vi "Calculate_Desired_Flowrates.vi"(4 "Atmos Pres (mbars)":dbl=1000.0 format="%.2f", 5 "Release temp (deg C)":dbl=20.0 format="%.2f", 6 "Density Ratio":string, 8 "Strength (% by volume)":dbl=3.0 format="%.2f", 9 "Stack Flowrate (l/min)":dbl=20.0 format="%.2f") -> (0 "Error Message":string, 1 "Trace Q l/min":dbl format="%.2f", 2 "Carrier 2 l/min":dbl format="%.2f", 3 "Carrier 1 l/min":dbl format="%.2f")   [LabVIEW 2010]
uses:
  Anemometry/Anemometry Sub Vis/Globals/Gas_management_global.vi
panel:
  # "-Carrier 1 only\n-Carrier 2 only\n-Enter Ratio"
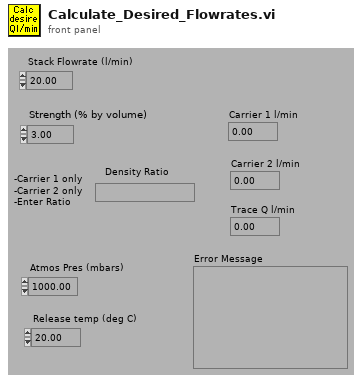
[diagram p1: front panel]
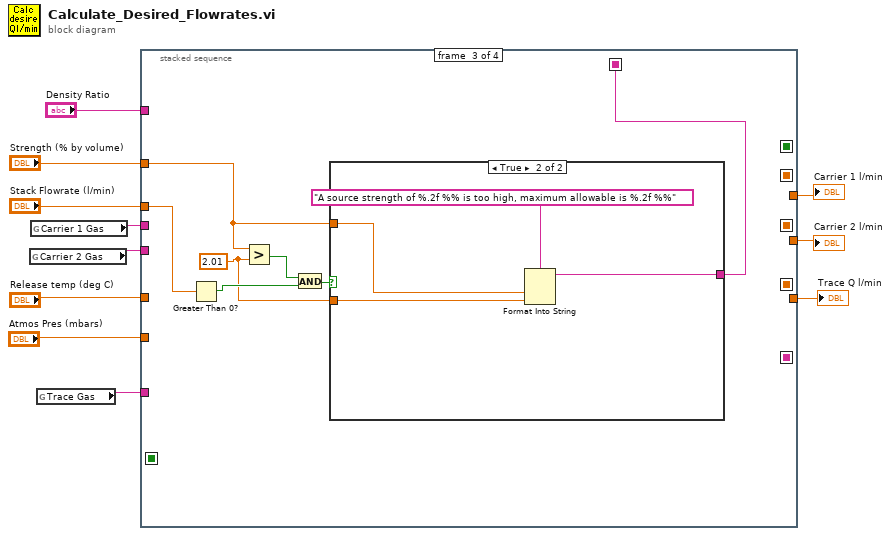
[diagram p0: block diagram]
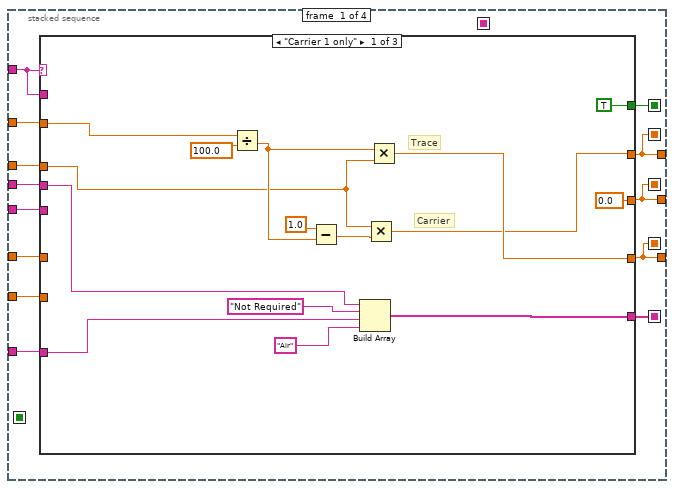
[diagram p2: hidden frame]
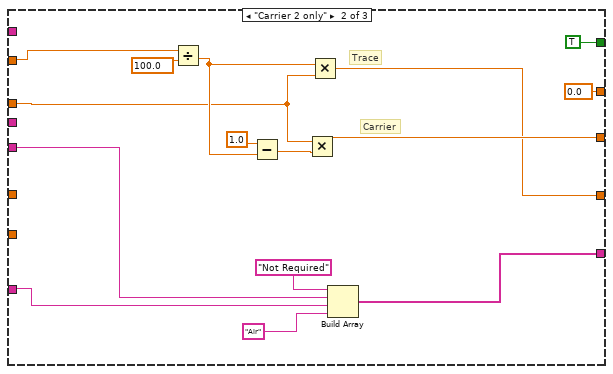
[diagram p3: hidden frame]
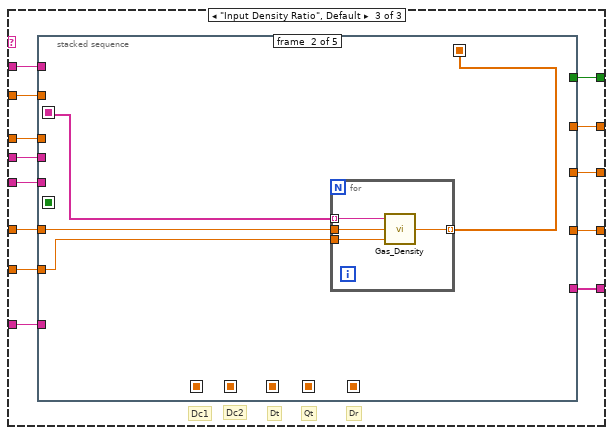
[diagram p4: hidden frame]
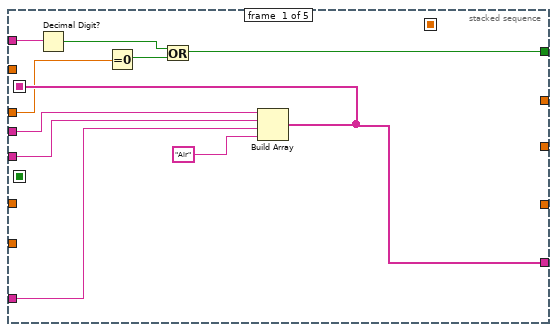
[diagram p5: hidden frame]
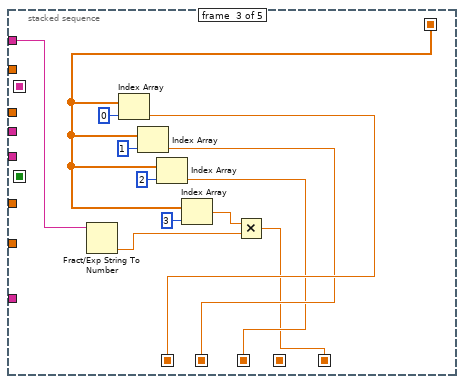
[diagram p6: hidden frame]
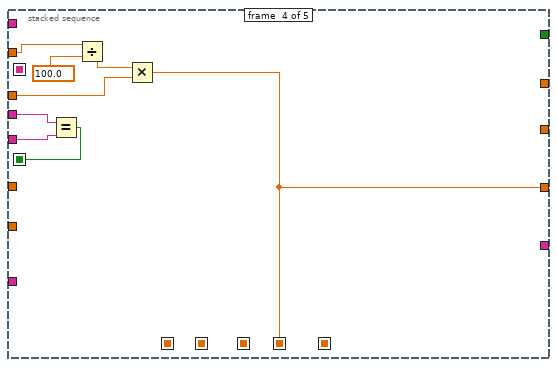
[diagram p7: hidden frame]
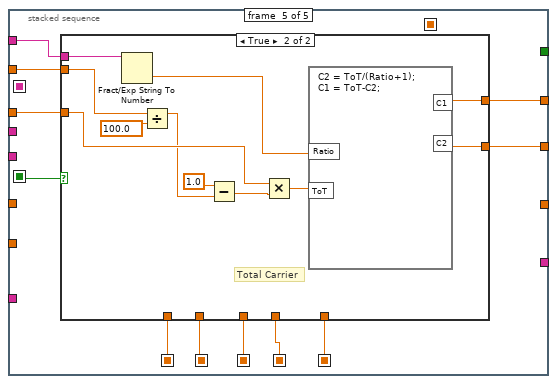
[diagram p8: hidden frame]
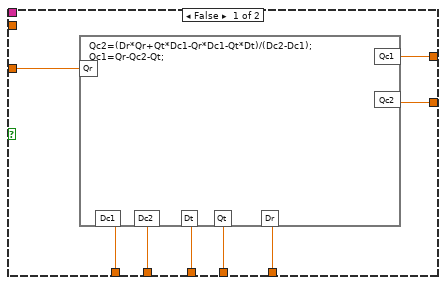
[diagram p9: hidden frame]
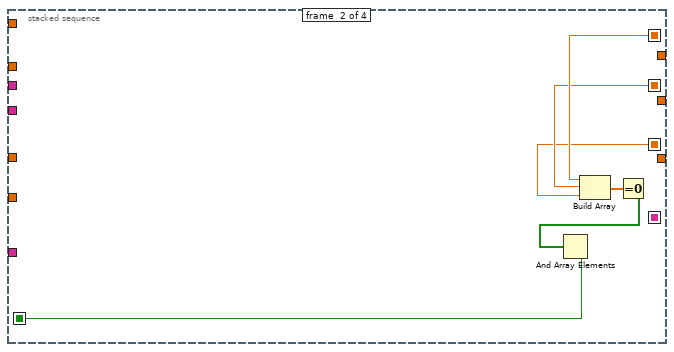
[diagram p10: hidden frame]
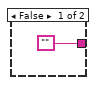
[diagram p11: hidden frame]
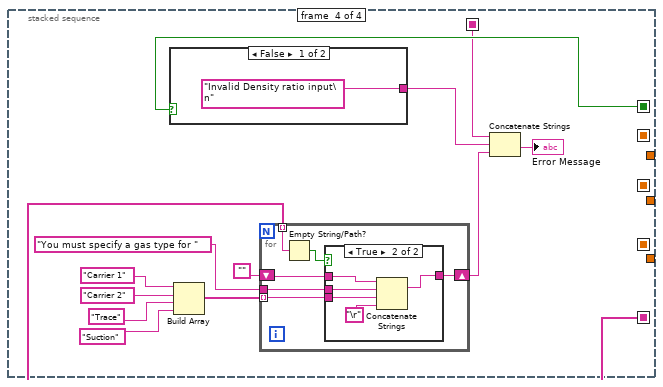
[diagram p12: hidden frame]
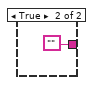
[diagram p13: hidden frame]
diagram:
  n1 = global read "Gas_management_global.vi" "Carrier 2 Gas"() -> (w2:string)
  n2 = global read "Gas_management_global.vi" "Carrier 1 Gas"() -> (w3:string)
  n3 = global read "Gas_management_global.vi" "Trace Gas"() -> (w1:string)
  n4 = stacked-sequence {
    seq-local: [w16 _ _ _] -> [_ _ _ w159]
    seq-local: [w15 _ _ _] -> [_ _ _ w158]
    seq-local: [w12 _ _ _] -> [_ w141 _ _]
    seq-local: [w13 _ _ _] -> [_ w140 _ _]
    seq-local: [w14 _ _ _] -> [_ w139 _ _]
    seq-local: [_ w136 _ _] -> [_ _ _ _]
    seq-local: [_ _ w142 _] -> [_ _ _ w154]
    tunnel: "Release temp (deg C)" -> [w24 _ _ _]
    tunnel: "Atmos Pres (mbars)" -> [w23 _ _ _]
    tunnel: "Stack Flowrate (l/min)" -> [w22 _ w148 _]
    tunnel: "Strength (% by volume)" -> [w21 _ w143 _]
    tunnel: [w14 _ _ _] -> w7
    tunnel: [w12 _ _ _] -> w6
    tunnel: [w13 _ _ _] -> w5
    tunnel: "Density Ratio" -> [w20 _ _ _]
    tunnel: w3 -> [w19 _ _ _]
    tunnel: w2 -> [w18 _ _ _]
    tunnel: w1 -> [w17 _ _ _]
    frame #0 {
      n5 = case shown="\"Carrier 1 only\"" w20 {
        tunnel: w24 -> [_ _ w67]
        tunnel: w23 -> [_ _ w66]
        tunnel: w22 -> [w33 w50 w65]
        tunnel: w21 -> [w36 w49 w64]
        tunnel: [0.0 ("Qc2") w48 w63] -> w13
        tunnel: [w34 w47 w62] -> w14
        tunnel: [w32 0.0 ("Qc1") w61] -> w12
        tunnel: w20 -> [_ _ w60]
        tunnel: w19 -> [w28 _ w59]
        tunnel: w18 -> [_ w43 w58]
        tunnel: w17 -> [w27 w42 w57]
        tunnel: [w26 w41 w56] -> w16
        tunnel: [TRUE TRUE w55] -> w15
        frame "Carrier 1 only" {
          # "Carrier"
          # "Trace"
          n6 = Divide(x=w36, y=100.0) -> (x/y=w35:dbl)
          n7 = Subtract(x=1.0, y=w35) -> (x-y=w39:dbl)
          n8 = Build Array(w28, "Not Required" ("Input Element"), w27, "Air") -> (w26:string[])
          n9 = Multiply(x=w33, y=w39) -> (x*y=w32:dbl)
          n10 = Multiply(x=w35, y=w33) -> (x*y=w34:dbl)
        }
        frame "Carrier 2 only" {
          # "Carrier"
          # "Trace"
          n11 = Divide(x=w49, y=100.0) -> (x/y=w51:dbl)
          n12 = Subtract(x=1.0, y=w51) -> (x-y=w54:dbl)
          n13 = Multiply(x=w50, y=w54) -> (x*y=w48:dbl)
          n14 = Multiply(x=w51, y=w50) -> (x*y=w47:dbl)
          n15 = Build Array("Not Required" ("Input Element"), w43, w42, "Air") -> (w41:string[])
        }
        frame "Input Density Ratio", Default {
          # "Dr"
          # "Qt"
          # "Dt"
          # "Dc2"
          # "Dc1"
          n16 = stacked-sequence {
            seq-local: [_ _ w92 _ _] -> [_ _ _ _ w116]
            seq-local: [_ _ w91 _ _] -> [_ _ _ _ w115]
            seq-local: [_ _ w90 _ _] -> [_ _ _ _ w114]
            seq-local: [_ _ _ w101 _] -> [_ _ _ _ w113]
            seq-local: [_ w79 _ _ _] -> [_ _ w93 _ _]
            seq-local: [_ _ w88 _ _] -> [_ _ _ _ w109]
            seq-local: [w72 _ _ _ _] -> [_ w78 _ _ _]
            seq-local: [_ _ _ w98 _] -> [_ _ _ _ w108]
            tunnel: w67 -> [_ w81 _ _ _]
            tunnel: w66 -> [_ w80 _ _ _]
            tunnel: w65 -> [w71 _ _ w104 w112]
            tunnel: w64 -> [_ _ _ w102 w106]
            tunnel: [_ _ _ _ w110] -> w63
            tunnel: [_ _ _ w101 _] -> w62
            tunnel: [_ _ _ _ w111] -> w61
            tunnel: w60 -> [w73 _ w87 _ w107]
            tunnel: w59 -> [w76 _ _ w100 _]
            tunnel: w58 -> [w75 _ _ w99 _]
            tunnel: w57 -> [w74 _ _ _ _]
            tunnel: [w72 _ _ _ _] -> w56
            tunnel: [w68 _ _ _ _] -> w55
            frame #0 {
              n17 = Decimal Digit?(1:w73) -> (0:w70:bool)
              n18 = Equal To 0?(x=w71) -> (x = 0?=w69:bool)
              n19 = Or(x=w70, y=w69) -> (x .or. y?=w68:bool)
              n20 = Build Array(w76, w75, w74, "Air") -> (w72:string[])
            }
            frame #1 {
              n21 = for {
                tunnel: w81 -> [w85]
                tunnel: w80 -> [w84]
                tunnel: [w83] -> w79 mode=indexing
                tunnel: w78 -> [w82] mode=indexing
                n22 = call "Gas_Density.vi"("Pressure (mbars)"=w84, "Temperature (deg C)"=w85, "Gas Name"=w82) -> ("Density Kg/m3"=w83:dbl)
              }
            }
            frame #2 {
              n23 = Fract/Exp String To Number(string=w87) -> (number=w86:dbl)  [unwired: 4 out]
              n24 = Index Array(array=w93, index=0 ("Index")) -> (element=w92:dbl)
              n25 = Index Array(array=w93, index=1 ("Index")) -> (element=w91:dbl)
              n26 = Index Array(array=w93, index=2 ("Index")) -> (element=w90:dbl)
              n27 = Index Array(array=w93, index=3 ("Index")) -> (element=w89:dbl)
              n28 = Multiply(x=w89, y=w86) -> (x*y=w88:dbl)
            }
            frame #3 {
              n29 = Equal?(x=w100, y=w99) -> (x = y?=w98:bool)
              n30 = Divide(x=w102, y=100.0) -> (x/y=w103:dbl)
              n31 = Multiply(x=w103, y=w104) -> (x*y=w101:dbl)
            }
            frame #4 {
              n32 = case shown="True" w108 {
                tunnel: w116 -> [w124 _]
                tunnel: w115 -> [w123 _]
                tunnel: w114 -> [w122 _]
                tunnel: w113 -> [w121 _]
                tunnel: w112 -> [w120 w130]
                tunnel: [w119 w125] -> w111
                tunnel: [w118 w126] -> w110
                tunnel: w109 -> [w117 _]
                tunnel: w107 -> [_ w135]
                tunnel: w106 -> [_ w131]
                frame False {
                  n33 = formula code="Qc2=(Dr*Qr+Qt*Dc1-Qr*Dc1-Qt*Dt)/(Dc2-Dc1);\nQc1=Qr-Qc2-Qt;"("Dc1"=w124, "Dc2"=w123, "Dt"=w122, "Qt"=w121, "Dr"=w117, "Qr"=w120) -> ("Qc2"=w118:dbl, "Qc1"=w119:dbl)
                }
                frame True {
                  # "Total Carrier"
                  n34 = Fract/Exp String To Number(string=w135) -> (number=w127:dbl)  [unwired: 4 out]
                  n35 = Divide(x=w131, y=100.0) -> (x/y=w129:dbl)
                  n36 = Subtract(x=1.0, y=w129) -> (x-y=w134:dbl)
                  n37 = Multiply(x=w130, y=w134) -> (x*y=w128:dbl)
                  n38 = formula code="C2 = ToT/(Ratio+1);\nC1 = ToT-C2;"("ToT"=w128, "Ratio"=w127) -> ("C1"=w125:dbl, "C2"=w126:dbl)
                }
              }
            }
          }
        }
      }
    }
    frame #1 {
      n39 = Build Array(w141, w140, w139) -> (w138:dbl[])
      n40 = Equal To 0?(x=w138) -> (x = 0?=w137:bool[])
      n41 = And Array Elements(Boolean array=w137) -> (logical AND=w136:bool)
    }
    frame #2 {
      w144 = 2.01 ("y")
      n42 = Greater Than 0?(x=w148) -> (x > 0?=w146:bool)
      n43 = Greater?(x=w143, y=w144) -> (0:w147:bool)
      n44 = And(x=w147, y=w146) -> (x .and. y?=w145:bool)
      n45 = case shown="True" w145 {
        tunnel: w143 -> [_ w153]
        tunnel: w144 -> [_ w151]
        tunnel: ["" w150] -> w142
        frame False {
        }
        frame True {
          n46 = Format Into String(format string="A source strength of %.2f %% is too high, maximum allowable is %.2f %%" ("Format String"), w153, w151) -> (resulting string=w150:string)  [unwired: 2 in, 1 out]
        }
      }
    }
    frame #3 {
      n47 = case shown="False" w158 {
        tunnel: ["Invalid Density ratio input\n" ""] -> w156
        frame False {
        }
        frame True {
        }
      }
      n48 = Build Array("Carrier 1" ("Gas Line Name"), "Carrier 2" ("Gas Line Name"), "Trace" ("Gas Line Name"), "Suction" ("Gas Line Name")) -> (w161:string[])
      n49 = for {
        shift-right: [w170] -> w157
        shift-left: "" -> [w171]
        tunnel: "You must specify a gas type for " -> [w173]
        tunnel: w161 -> [w172] mode=indexing
        tunnel: w159 -> [w169] mode=indexing
        n50 = Empty String/Path?(string/path=w169) -> (empty?=w174:bool)
        n51 = case shown="True" w174 {
          tunnel: w173 -> [_ w180]
          tunnel: w172 -> [_ w179]
          tunnel: w171 -> [w175 w178]
          tunnel: [w175 w177] -> w170
          frame False {
          }
          frame True {
            n52 = Concatenate Strings(w178, w180, w179, "\r") -> (w177:string)
          }
        }
      }
      n53 = Concatenate Strings(w154, w156, w157) -> (→"Error Message":string)
    }
  }
  "Carrier 1 l/min" <- w6
  "Carrier 2 l/min" <- w5
  "Trace Q l/min" <- w7
